vi "EncuentraJoystick.vi"() -> (0 "error out":errorcluster, 3 "Refnum out":refnum<k1>)   [LabVIEW 2014]
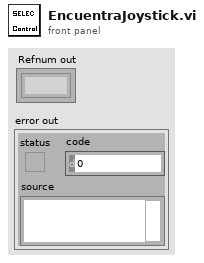
[diagram p1: front panel]
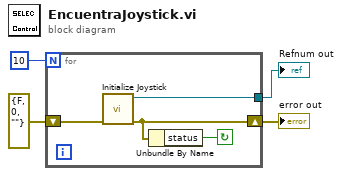
[diagram p0: block diagram]
diagram:
  n1 = for {
    N: 10 -> [_]
    shift-right: [w6] -> w3
    shift-left: errorcluster {"status"=FALSE, "code"=0, "source"=""} ("error out") -> [w8]
    tunnel: [w5] -> w2
    stop <- w7 continue-if-true
    n2 = call <vilib>:"Initialize Joystick.vi"("error in (no error)"=w8) -> ("error out"=w6:errorcluster, "device ID"=w5:refnum<k1>)  [unwired: 1 in, 8 out]
    n3 = Unbundle By Name(w6) -> ("status"=w7:bool)
  }
  "error out" <- w3
  "Refnum out" <- w2
